vi "LabVIEW_ArduinoControls8-12-21.vi"() -> ()   [LabVIEW 2020]
uses:
  <vilib>/Instr/_visa.llb/VISA Configure Serial Port (Instr).vi
panel:
  out "Vert Distance 2":dbl[](graph)
  out "Horz Distance":dbl[](graph)
  out "Average Temp":dbl[](graph)
  out "RPM":dbl[](graph)
  in  "DRILL STOP":bool
  in  "Drill Speed Arduino 2.0 Write Stop":bool
  in  "Slow Down":bool
  in  "Speed Up":bool
  in  "Drill Speed Arduino 2 Write":refnum<visa-resource-name>
  in  "Stepper Arduino 1 Serial Read":refnum<visa-resource-name>
  out "Weight on Bit A1":dbl[](graph)
  out "Vertical Motor Speed A1":dbl[](graph)
  out "Data Packet Arduini 1 Matched":i32
  in  "Arduino 1.0 Read Stop":bool
  in  "Arduino 2.0 Read Stop":bool
  in  "Emergency Stop! 3":bool
  in  "Emergency Stop! 2":bool
  in  "GO DOWN 3":bool
  in  "GO DOWN 2":bool
  in  "GO UP 3":bool
  in  "GO UP 2":bool
  in  "MAX SPEED 3":bool
  in  "MAX SPEED 2":bool
  in  "SLOWEST SPEED 3":bool
  in  "SLOWEST SPEED 2":bool
  in  "Decellerate 3":bool
  in  "Decellerate 2":bool
  in  "Accelerate 3":bool
  in  "Accelerate 2":bool
  in  "Drill Speed Arduino 2 Serial Read":refnum<visa-resource-name>
  out "Data Packet Received":i32
  out "Drill Amps A2":dbl[](graph)
  in  "GO UP":bool
  in  "GO DOWN":bool
  in  "MAX SPEED":bool
  in  "SLOWEST SPEED":bool
  out "System Amps A2":dbl[](graph)
  out "concatenated string":string
  in  "Arduino 1.0 Write Stop":bool
  in  "Emergency Stop!":bool
  in  "Decellerate":bool
  in  "Stepper Arduino 1 Write":refnum<visa-resource-name>
  in  "Accelerate":bool
  # "Drill Speed Controls"
  # "WINCH CONTROLS"
  # "VERTICAL STEPPER MOTOR CONTROLS"
  # "HORIZONTAL STEPPER MOTOR CONTROLS"
  # "-1 Means Not Found\nany value greater than 0 corresponds to the amount\nof matching characters found"
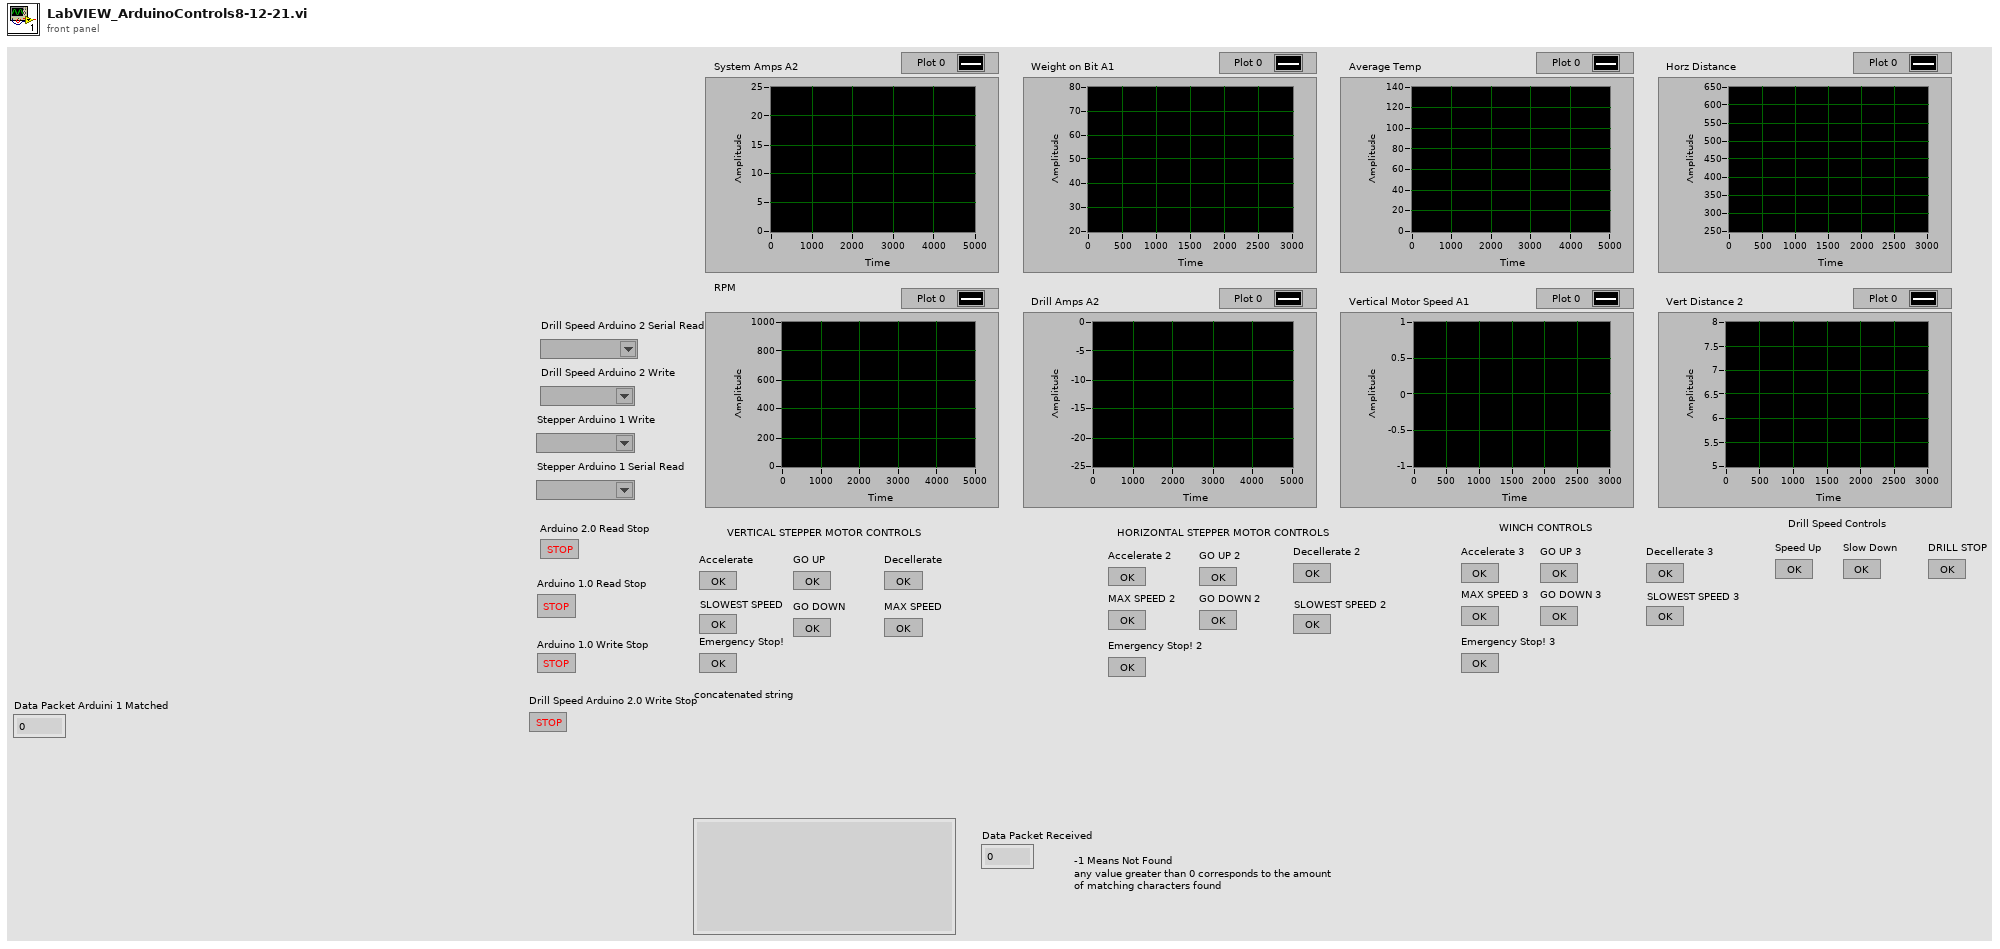
[diagram p1: front panel]
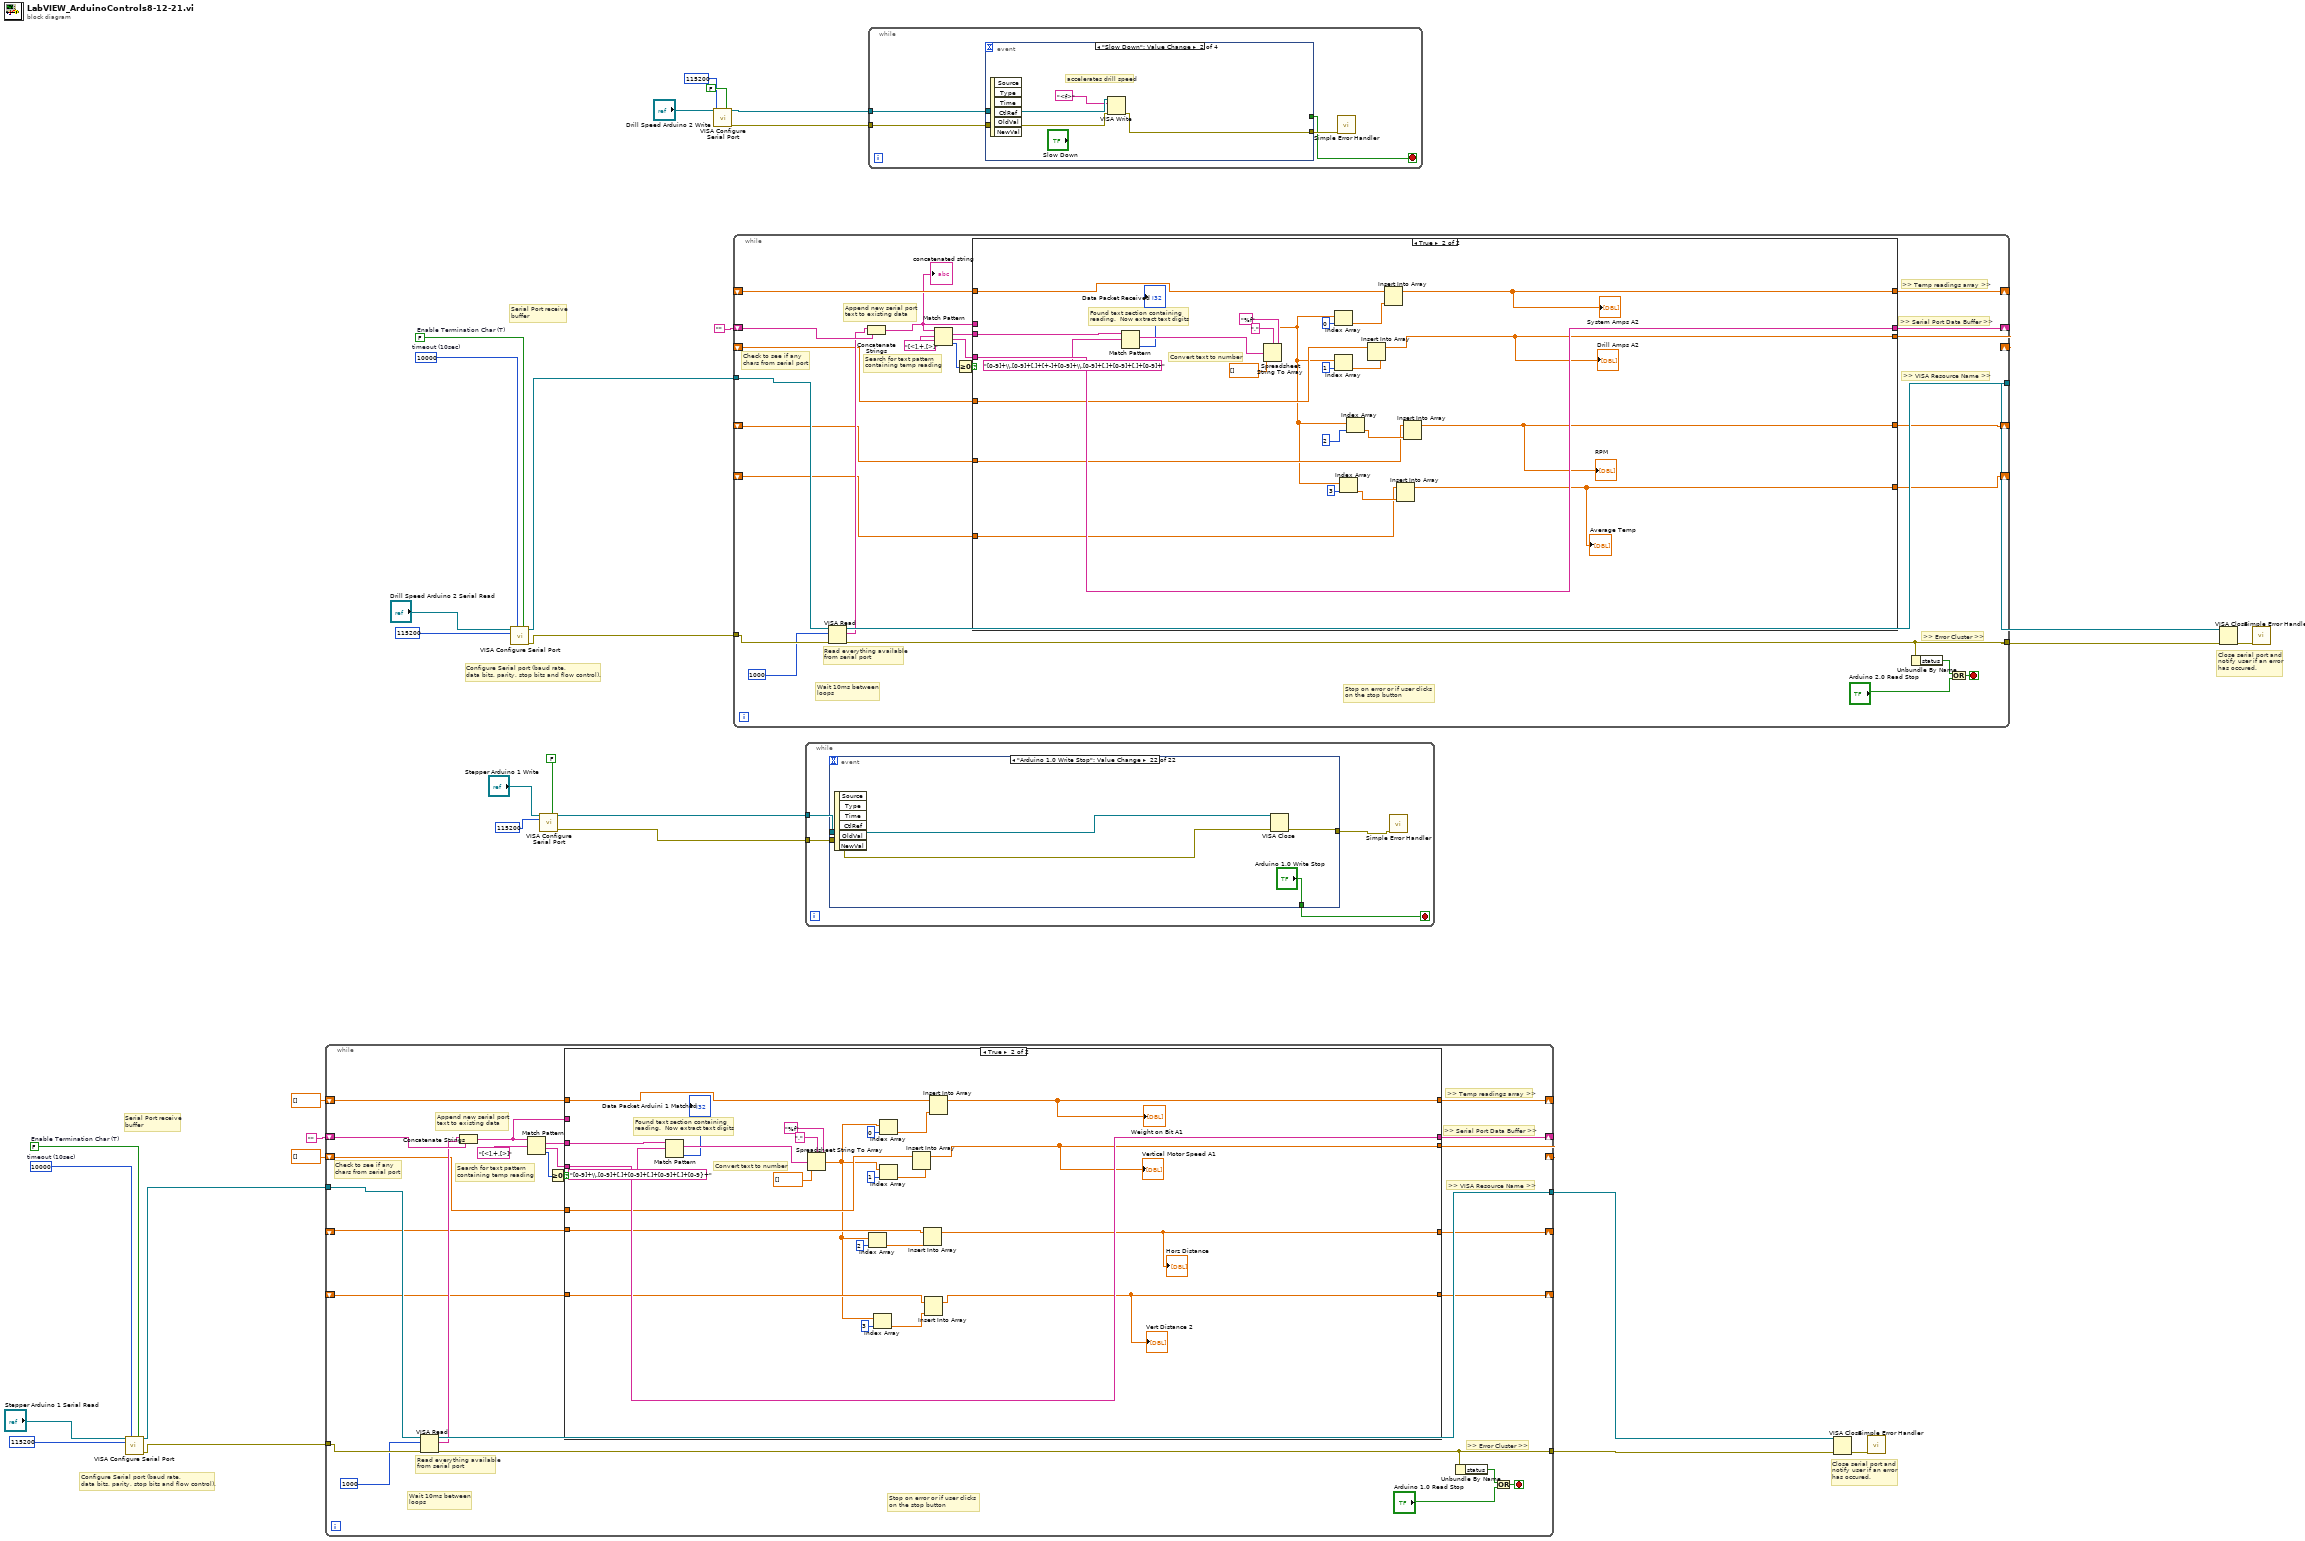
[diagram p0: block diagram]
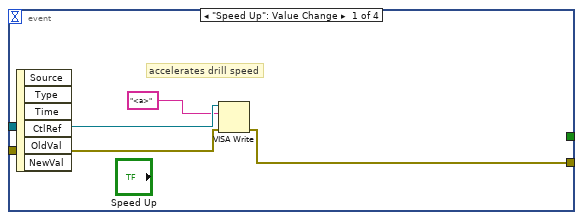
[diagram p2: hidden frame]
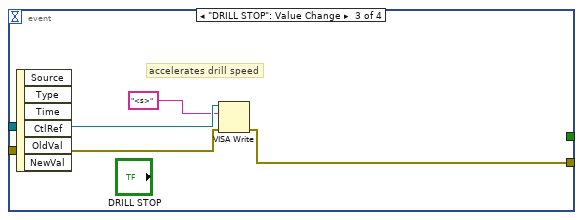
[diagram p3: hidden frame]
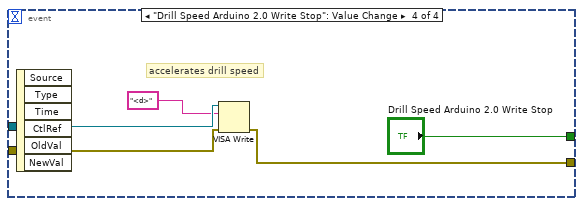
[diagram p4: hidden frame]
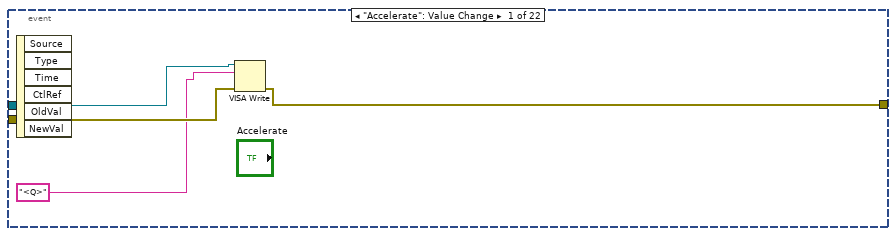
[diagram p7: hidden frame]
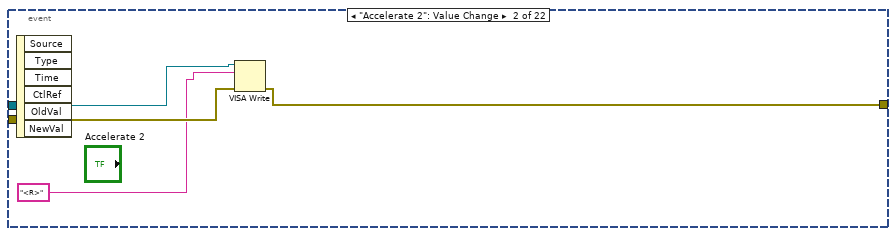
[diagram p8: hidden frame]
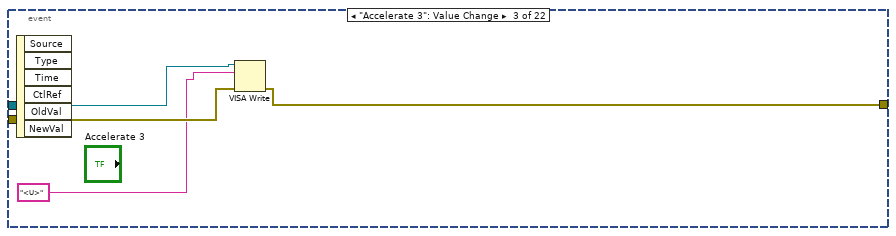
[diagram p9: hidden frame]
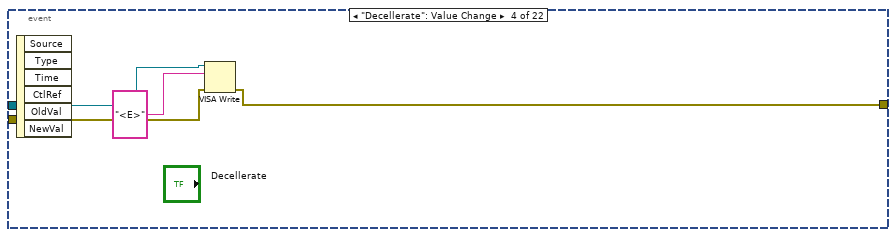
[diagram p10: hidden frame]
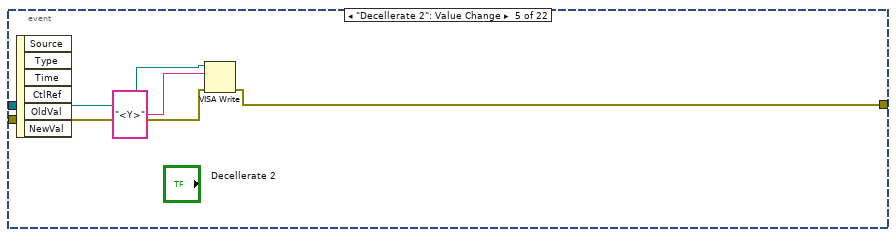
[diagram p11: hidden frame]
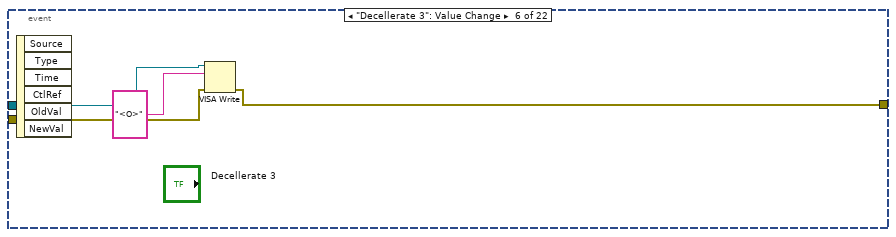
[diagram p12: hidden frame]
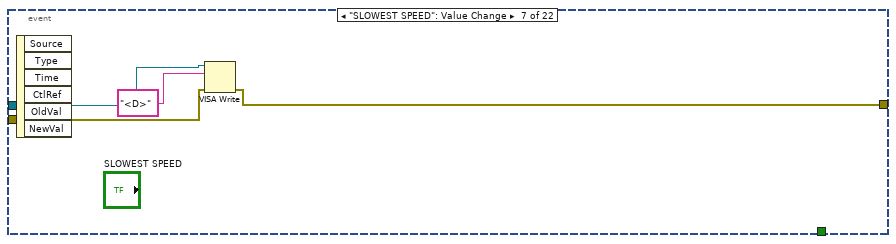
[diagram p13: hidden frame]
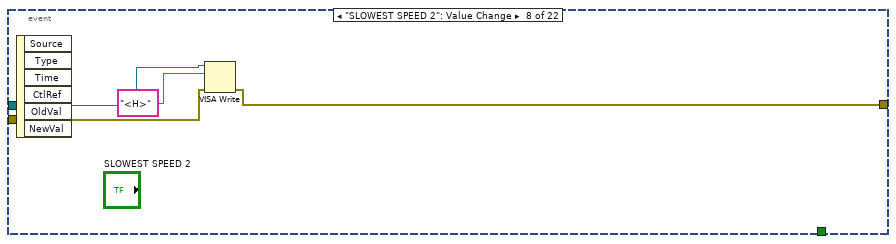
[diagram p14: hidden frame]
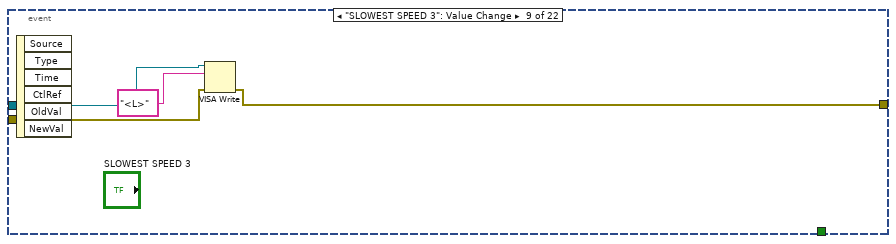
[diagram p15: hidden frame]
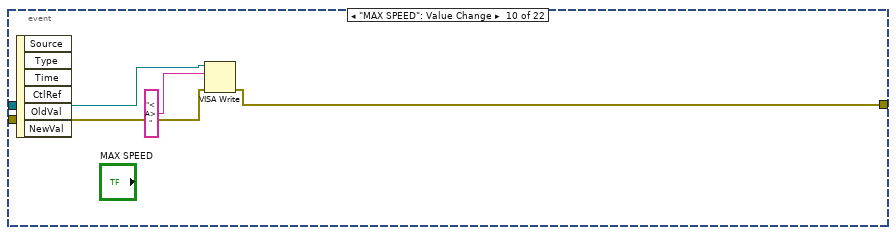
[diagram p16: hidden frame]
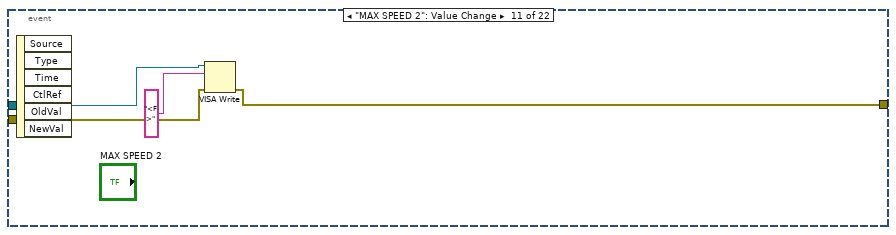
[diagram p17: hidden frame]
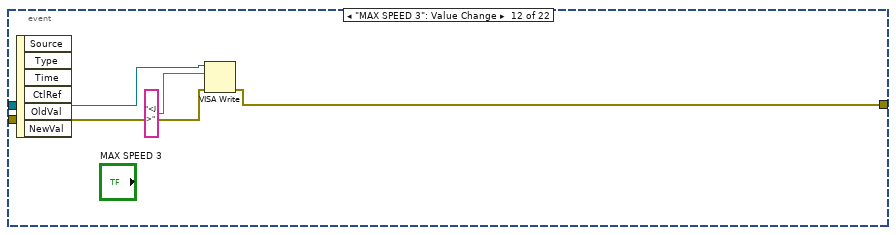
[diagram p18: hidden frame]
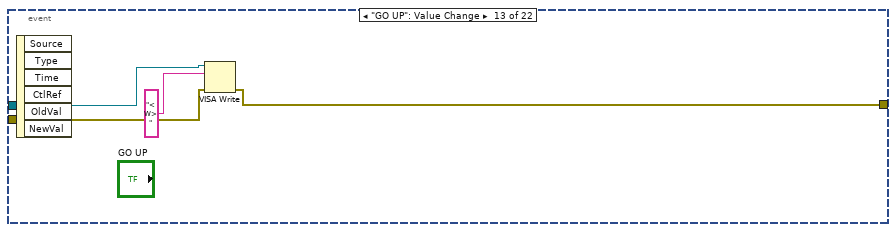
[diagram p19: hidden frame]
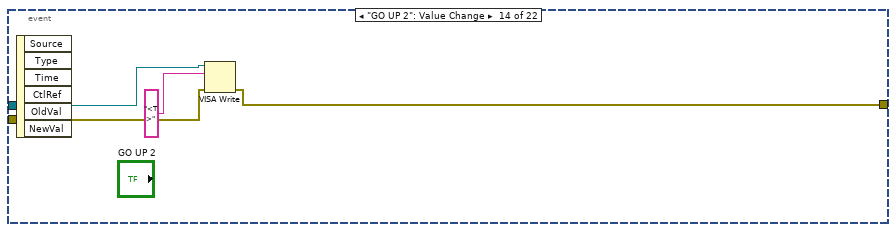
[diagram p20: hidden frame]
diagram:
  w13 = FALSE  # Enable Termination Char (T)
  w14 = u32 10000  # timeout (10sec)
  w24 = FALSE  # Enable Termination Char (T)
  w25 = u32 10000  # timeout (10sec)
  # "Close serial port and\nnotify user if an error\nhas occured."
  # "Serial Port receive\nbuffer"
  # "Configure Serial port (baud rate,\ndata bits, parity, stop bits and flow control)."
  # "Close serial port and\nnotify user if an error\nhas occured."
  # "Serial Port receive\nbuffer"
  # "Configure Serial port (baud rate,\ndata bits, parity, stop bits and flow control)."
  n1 = call-poly "VISA Configure Serial Port"("VISA resource name"="Stepper Arduino 1 Serial Read", "timeout (10sec)"=w14, "Enable Termination\nChar (T)"=w13, "baud rate (9600)"=u32 115200) -> ("VISA resource name out"=w10:refnum<visa-resource-name>, "error out"=w9:errorcluster)  [unwired: 10 in]
  n2 = while {
    tunnel: [w55] -> w17
    tunnel: [w57] -> w16
    shift-right: [w50] -> _
    shift-left: "" -> [w56]
    shift-right: [w52] -> _
    shift-left: dbl[] [] -> [w51]
    tunnel: w10 -> [w49]
    tunnel: w9 -> [w48]
    shift-right: [w40] -> _
    shift-left: dbl[] [] -> [w39]
    shift-right: [w35] -> _
    shift-left: _ -> [w36]
    shift-right: [w33] -> _
    shift-left: _ -> [w34]
    stop <- w54 stop-if-true
    # "Search for text pattern\ncontaining temp reading"
    # "Append new serial port\ntext to existing data"
    # "Read everything available\nfrom serial port"
    # "Wait 10ms between \nloops"
    # "Stop on error or if user clicks \non the stop button"
    # ">> Error Cluster >>"
    # ">> VISA Resource Name >>"
    # ">> Temp readings array >>"
    # ">> Serial Port Data Buffer >>"
    # "Check to see if any\nchars from serial port"
    n3 = VISA Read(VISA resource name=w49, byte count=u32 1000, error in (no error)=w48) -> (VISA resource name out=w57:refnum<visa-resource-name>, read buffer=w42:string, error out=w55:errorcluster)  [unwired: 1 out]
    n4 = Concatenate Strings(w42, w56) -> (w37:string)
    n5 = Match Pattern(string=w37, regular expression="[<].+.[>]") -> (match substring=w44:string, after substring=w43:string, offset past match=w46:i32)  [unwired: 1 in, 1 out]
    n6 = Greater Or Equal To 0?(x=w46) -> (x >= 0?=w45:bool)
    n7 = case shown="True" w45 {
      tunnel: w44 -> [_ w86]
      tunnel: w43 -> [_ w87]
      tunnel: [w60 w87] -> w50
      tunnel: [w62 w84] -> w52
      tunnel: w51 -> [w62 w72]
      tunnel: [w61 w75] -> w40
      tunnel: w39 -> [w61 w76]
      tunnel: w37 -> [w60 _]
      tunnel: w36 -> [w59 w70]
      tunnel: [w59 w68] -> w35
      tunnel: w34 -> [w58 w66]
      tunnel: [w58 w63] -> w33
      frame False {
        # "Did not find text pattern in the buffer.  Try again in the next loop after new data \nhas been received."
      }
      frame True {
        # "Convert text to number"
        # "Found text section containing \nreading.  Now extract text digits"
        n8 = Match Pattern(string=w86, regular expression="[0-9]+\\.[0-9]+[,]+[0-9]+[,]+[0-9]+[,]+[0-9}+") -> (match substring=w79:string, offset past match=→"Data Packet Arduini 1 Matched":i32)  [unwired: 1 in, 2 out]
        n9 = Spreadsheet String To Array(delimiter (Tab)=",", format string="%f", spreadsheet string=w79, array type (2D Dbl)=dbl[] []) -> (array=w65:dbl[])
        n10 = Index Array(array=w65, index=2) -> (element=w71:dbl)
        n11 = Index Array(array=w65, index=3) -> (element=w67:dbl)
        n12 = Index Array(array=w65, index=0 ("index (row)")) -> (element=w78:dbl)
        n13 = Index Array(array=w65, index=1 ("index (row)")) -> (element=w77:dbl)
        n14 = Insert Into Array(array=w76, new element=w77) -> (w75:dbl[])  [unwired: 1 in]
        "Vertical Motor Speed A1" <- w75
        n15 = Insert Into Array(array=w70, new element=w71) -> (w68:dbl[])  [unwired: 1 in]
        "Horz Distance" <- w68
        n16 = Insert Into Array(array=w66, new element=w67) -> (w63:dbl[])  [unwired: 1 in]
        "Vert Distance 2" <- w63
        n17 = Insert Into Array(array=w72, new element=w78) -> (w84:dbl[])  [unwired: 1 in]
        "Weight on Bit A1" <- w84
      }
    }
    n18 = Unbundle By Name(w55) -> ("status"=w53:bool)
    n19 = Or(x=w53, y="Arduino 1.0 Read Stop") -> (x .or. y?=w54:bool)
  }
  n20 = call-poly "VISA Configure Serial Port"("VISA resource name"="Drill Speed Arduino 2 Serial Read", "timeout (10sec)"=w25, "Enable Termination\nChar (T)"=w24, "baud rate (9600)"=u32 115200) -> ("VISA resource name out"=w21:refnum<visa-resource-name>, "error out"=w20:errorcluster)  [unwired: 10 in]
  n21 = call-poly "VISA Configure Serial Port"("VISA resource name"="Stepper Arduino 1 Write", "Enable Termination\nChar (T)"=FALSE ("Enable Termination\nChar (T)"), "baud rate (9600)"=u32 115200) -> ("VISA resource name out"=w32:refnum<visa-resource-name>, "error out"=w31:errorcluster)  [unwired: 11 in]
  n22 = call-poly "VISA Configure Serial Port"("VISA resource name"="Drill Speed Arduino 2 Write", "Enable Termination\nChar (T)"=FALSE ("Enable Termination\nChar (T)"), "baud rate (9600)"=u32 115200) -> ("VISA resource name out"=w7:refnum<visa-resource-name>, "error out"=w6:errorcluster)  [unwired: 11 in]
  n23 = while {
    tunnel: [w110] -> w28
    tunnel: [w112] -> w27
    shift-right: [w105] -> _
    shift-left: "" -> [w111]
    shift-right: [w107] -> _
    shift-left: _ -> [w106]
    tunnel: w21 -> [w104]
    tunnel: w20 -> [w103]
    shift-right: [w95] -> _
    shift-left: _ -> [w94]
    shift-right: [w90] -> _
    shift-left: _ -> [w91]
    shift-right: [w88] -> _
    shift-left: _ -> [w89]
    stop <- w109 stop-if-true
    # "Search for text pattern\ncontaining temp reading"
    # "Append new serial port\ntext to existing data"
    # "Read everything available\nfrom serial port"
    # "Wait 10ms between \nloops"
    # "Stop on error or if user clicks \non the stop button"
    # ">> Error Cluster >>"
    # ">> VISA Resource Name >>"
    # ">> Temp readings array >>"
    # ">> Serial Port Data Buffer >>"
    # "Check to see if any\nchars from serial port"
    n24 = VISA Read(VISA resource name=w104, byte count=u32 1000, error in (no error)=w103) -> (VISA resource name out=w112:refnum<visa-resource-name>, read buffer=w97:string, error out=w110:errorcluster)  [unwired: 1 out]
    n25 = Concatenate Strings(w97, w111) -> (w92:string)
    "concatenated string" <- w92
    n26 = Match Pattern(string=w92, regular expression="[<].+.[>]") -> (match substring=w99:string, after substring=w98:string, offset past match=w101:i32)  [unwired: 1 in, 1 out]
    n27 = Greater Or Equal To 0?(x=w101) -> (x >= 0?=w100:bool)
    n28 = case shown="True" w100 {
      tunnel: w99 -> [_ w141]
      tunnel: w98 -> [_ w142]
      tunnel: [w115 w142] -> w105
      tunnel: [w117 w139] -> w107
      tunnel: w106 -> [w117 w127]
      tunnel: [w116 w130] -> w95
      tunnel: w94 -> [w116 w131]
      tunnel: w92 -> [w115 _]
      tunnel: w91 -> [w114 w124]
      tunnel: [w114 w123] -> w90
      tunnel: w89 -> [w113 w119]
      tunnel: [w113 w118] -> w88
      frame False {
        # "Did not find text pattern in the buffer.  Try again in the next loop after new data \nhas been received."
      }
      frame True {
        # "Convert text to number"
        # "Found text section containing \nreading.  Now extract text digits"
        n29 = Match Pattern(string=w141, regular expression="[0-9]+\\.[0-9]+[,]+[+-]+[0-9]+\\.[0-9]+[,]+[0-9]+[,]+[0-9]+") -> (match substring=w134:string, offset past match=→"Data Packet Received":i32)  [unwired: 1 in, 2 out]
        n30 = Spreadsheet String To Array(delimiter (Tab)=",", format string="%f", spreadsheet string=w134, array type (2D Dbl)=dbl[] []) -> (array=w120:dbl[])
        n31 = Index Array(array=w120, index=0 ("index (row)")) -> (element=w133:dbl)
        n32 = Index Array(array=w120, index=1 ("index (row)")) -> (element=w132:dbl)
        n33 = Index Array(array=w120, index=3) -> (element=w122:dbl)
        n34 = Index Array(array=w120, index=2) -> (element=w125:dbl)
        n35 = Insert Into Array(array=w131, new element=w132) -> (w130:dbl[])  [unwired: 1 in]
        "Drill Amps A2" <- w130
        n36 = Insert Into Array(array=w127, new element=w133) -> (w139:dbl[])  [unwired: 1 in]
        "System Amps A2" <- w139
        n37 = Insert Into Array(array=w119, new element=w122) -> (w118:dbl[])  [unwired: 1 in]
        "Average Temp" <- w118
        n38 = Insert Into Array(array=w124, new element=w125) -> (w123:dbl[])  [unwired: 1 in]
        "RPM" <- w123
      }
    }
    n39 = Unbundle By Name(w110) -> ("status"=w108:bool)
    n40 = Or(x=w108, y="Arduino 2.0 Read Stop") -> (x .or. y?=w109:bool)
  }
  n41 = while {
    tunnel: w32 -> [w146]
    tunnel: w31 -> [w145]
    stop <- w143 stop-if-true
    n42 = event shown="[21] \"Arduino 1.0 Write Stop\": Value Change" {
      selector: _ -> [_ _ _ _ _ _ _ _ _ _ _ _ _ _ _ _ _ _ _ _ _ _]
      dyn-events: _ -> [_ _ _ _ _ _ _ _ _ _ _ _ _ _ _ _ _ _ _ _ _ _]
      timeout: _ -> [_ _ _ _ _ _ _ _ _ _ _ _ _ _ _ _ _ _ _ _ _ _]
      tunnel: [w150 w154 w158 w162 w166 w170 w174 w178 w182 w186 w190 w194 w198 w202 w206 w210 w214 w218 w222 w226 w230 w234] -> w144
      tunnel: w146 -> [w149 w153 w157 w160 w164 w168 w172 w176 w180 w184 w188 w192 w196 w200 w204 w208 w212 w216 w220 w224 w228 w233]
      tunnel: w145 -> [w148 w152 w156 w159 w163 w167 w171 w175 w179 w183 w187 w191 w195 w199 w203 w207 w211 w215 w219 w223 w227 w232]
      tunnel: [_ _ _ _ _ _ _ _ _ _ _ _ _ _ _ _ _ _ _ _ _ "Arduino 1.0 Write Stop"] -> w143
      event "Accelerate": Value Change {
        n43 = event-data() -> ()  [unwired: 1 in, 6 out]
        n44 = VISA Write(VISA resource name=w149, write buffer="<Q>", error in (no error)=w148) -> (error out=w150:errorcluster)  [unwired: 2 out]
      }
      event "Accelerate 2": Value Change {
        n45 = event-data() -> ()  [unwired: 1 in, 6 out]
        n46 = VISA Write(VISA resource name=w153, write buffer="<R>", error in (no error)=w152) -> (error out=w154:errorcluster)  [unwired: 2 out]
      }
      event "Accelerate 3": Value Change {
        n47 = event-data() -> ()  [unwired: 1 in, 6 out]
        n48 = VISA Write(VISA resource name=w157, write buffer="<U>", error in (no error)=w156) -> (error out=w158:errorcluster)  [unwired: 2 out]
      }
      event "Decellerate": Value Change {
        n49 = event-data() -> ()  [unwired: 1 in, 6 out]
        n50 = VISA Write(VISA resource name=w160, write buffer="<E>", error in (no error)=w159) -> (error out=w162:errorcluster)  [unwired: 2 out]
      }
      event "Decellerate 2": Value Change {
        n51 = event-data() -> ()  [unwired: 1 in, 6 out]
        n52 = VISA Write(VISA resource name=w164, write buffer="<Y>", error in (no error)=w163) -> (error out=w166:errorcluster)  [unwired: 2 out]
      }
      event "Decellerate 3": Value Change {
        n53 = event-data() -> ()  [unwired: 1 in, 6 out]
        n54 = VISA Write(VISA resource name=w168, write buffer="<O>", error in (no error)=w167) -> (error out=w170:errorcluster)  [unwired: 2 out]
      }
      event "SLOWEST SPEED": Value Change {
        n55 = event-data() -> ()  [unwired: 1 in, 6 out]
        n56 = VISA Write(VISA resource name=w172, write buffer="<D>", error in (no error)=w171) -> (error out=w174:errorcluster)  [unwired: 2 out]
      }
      event "SLOWEST SPEED 2": Value Change {
        n57 = event-data() -> ()  [unwired: 1 in, 6 out]
        n58 = VISA Write(VISA resource name=w176, write buffer="<H>", error in (no error)=w175) -> (error out=w178:errorcluster)  [unwired: 2 out]
      }
      event "SLOWEST SPEED 3": Value Change {
        n59 = event-data() -> ()  [unwired: 1 in, 6 out]
        n60 = VISA Write(VISA resource name=w180, write buffer="<L>", error in (no error)=w179) -> (error out=w182:errorcluster)  [unwired: 2 out]
      }
      event "MAX SPEED": Value Change {
        n61 = event-data() -> ()  [unwired: 1 in, 6 out]
        n62 = VISA Write(VISA resource name=w184, write buffer="<A>", error in (no error)=w183) -> (error out=w186:errorcluster)  [unwired: 2 out]
      }
      event "MAX SPEED 2": Value Change {
        n63 = event-data() -> ()  [unwired: 1 in, 6 out]
        n64 = VISA Write(VISA resource name=w188, write buffer="<F>", error in (no error)=w187) -> (error out=w190:errorcluster)  [unwired: 2 out]
      }
      event "MAX SPEED 3": Value Change {
        n65 = event-data() -> ()  [unwired: 1 in, 6 out]
        n66 = VISA Write(VISA resource name=w192, write buffer="<J>", error in (no error)=w191) -> (error out=w194:errorcluster)  [unwired: 2 out]
      }
      event "GO UP": Value Change {
        n67 = event-data() -> ()  [unwired: 1 in, 6 out]
        n68 = VISA Write(VISA resource name=w196, write buffer="<W>", error in (no error)=w195) -> (error out=w198:errorcluster)  [unwired: 2 out]
      }
      event "GO UP 2": Value Change {
        n69 = event-data() -> ()  [unwired: 1 in, 6 out]
        n70 = VISA Write(VISA resource name=w200, write buffer="<T>", error in (no error)=w199) -> (error out=w202:errorcluster)  [unwired: 2 out]
      }
      event "GO UP 3": Value Change {
        n71 = event-data() -> ()  [unwired: 1 in, 6 out]
        n72 = VISA Write(VISA resource name=w204, write buffer="<I>", error in (no error)=w203) -> (error out=w206:errorcluster)  [unwired: 2 out]
      }
      event "GO DOWN": Value Change {
        n73 = event-data() -> ()  [unwired: 1 in, 6 out]
        n74 = VISA Write(VISA resource name=w208, write buffer="<S>", error in (no error)=w207) -> (error out=w210:errorcluster)  [unwired: 2 out]
      }
      event "GO DOWN 2": Value Change {
        n75 = event-data() -> ()  [unwired: 1 in, 6 out]
        n76 = VISA Write(VISA resource name=w212, write buffer="<G>", error in (no error)=w211) -> (error out=w214:errorcluster)  [unwired: 2 out]
      }
      event "GO DOWN 3": Value Change {
        n77 = event-data() -> ()  [unwired: 1 in, 6 out]
        n78 = VISA Write(VISA resource name=w216, write buffer="<K>", error in (no error)=w215) -> (error out=w218:errorcluster)  [unwired: 2 out]
      }
      event "Emergency Stop!": Value Change {
        n79 = event-data() -> ()  [unwired: 1 in, 6 out]
        n80 = VISA Write(VISA resource name=w220, write buffer="<Z>", error in (no error)=w219) -> (error out=w222:errorcluster)  [unwired: 2 out]
      }
      event "Emergency Stop! 2": Value Change {
        n81 = event-data() -> ()  [unwired: 1 in, 6 out]
        n82 = VISA Write(VISA resource name=w224, write buffer="<C>", error in (no error)=w223) -> (error out=w226:errorcluster)  [unwired: 2 out]
      }
      event "Emergency Stop! 3": Value Change {
        n83 = event-data() -> ()  [unwired: 1 in, 6 out]
        n84 = VISA Write(VISA resource name=w228, write buffer="<N>", error in (no error)=w227) -> (error out=w230:errorcluster)  [unwired: 2 out]
      }
      event "Arduino 1.0 Write Stop": Value Change {
        n85 = event-data() -> ()  [unwired: 1 in, 6 out]
        n86 = VISA Close(VISA resource name=w233, error in (no error)=w232) -> (error out=w234:errorcluster)
      }
    }
    n87 = call <vilib>:"Simple Error Handler.vi"("error in (no error)"=w144) -> ()  [unwired: 4 in, 5 out]
  }
  n88 = while {
    tunnel: w7 -> [w238]
    tunnel: w6 -> [w237]
    stop <- w235 stop-if-true
    n89 = event shown="[1] \"Slow Down\": Value Change" {
      selector: _ -> [_ _ _ _]
      dyn-events: _ -> [_ _ _ _]
      timeout: _ -> [_ _ _ _]
      tunnel: w238 -> [w242 w246 w250 w255]
      tunnel: w237 -> [w241 w245 w249 w254]
      tunnel: [w239 w243 w247 w252] -> w236
      tunnel: [_ _ _ "Drill Speed Arduino 2.0 Write Stop"] -> w235
      event "Speed Up": Value Change {
        # "accelerates drill speed"
        n90 = event-data() -> ()  [unwired: 1 in, 6 out]
        n91 = VISA Write(VISA resource name=w242, write buffer="<a>", error in (no error)=w241) -> (error out=w239:errorcluster)  [unwired: 2 out]
      }
      event "Slow Down": Value Change {
        # "accelerates drill speed"
        n92 = event-data() -> ()  [unwired: 1 in, 6 out]
        n93 = VISA Write(VISA resource name=w246, write buffer="<f>", error in (no error)=w245) -> (error out=w243:errorcluster)  [unwired: 2 out]
      }
      event "DRILL STOP": Value Change {
        # "accelerates drill speed"
        n94 = event-data() -> ()  [unwired: 1 in, 6 out]
        n95 = VISA Write(VISA resource name=w250, write buffer="<s>", error in (no error)=w249) -> (error out=w247:errorcluster)  [unwired: 2 out]
      }
      event "Drill Speed Arduino 2.0 Write Stop": Value Change {
        # "accelerates drill speed"
        n96 = event-data() -> ()  [unwired: 1 in, 6 out]
        n97 = VISA Write(VISA resource name=w255, write buffer="<d>", error in (no error)=w254) -> (error out=w252:errorcluster)  [unwired: 2 out]
      }
    }
    n98 = call <vilib>:"Simple Error Handler.vi"("error in (no error)"=w236) -> ()  [unwired: 4 in, 5 out]
  }
  n99 = VISA Close(VISA resource name=w16, error in (no error)=w17) -> (error out=w15:errorcluster)
  n100 = call <vilib>:"Simple Error Handler.vi"("error in (no error)"=w15) -> ()  [unwired: 4 in, 5 out]
  n101 = VISA Close(VISA resource name=w27, error in (no error)=w28) -> (error out=w26:errorcluster)
  n102 = call <vilib>:"Simple Error Handler.vi"("error in (no error)"=w26) -> ()  [unwired: 4 in, 5 out]
